vi "Read Search.vi"(11 "DiagramObject in":refnum<class "DiagramObject.lvclass">) -> (2 "Search":refnum<class "Search.lvclass">, 3 "DiagramObject out":refnum<class "DiagramObject.lvclass">)   [LabVIEW 2016, in "DiagramObject.lvclass"]
uses:
  DiagramObject.lvclass
  Search/Search.lvclass
  DiagramObject.lvclass/DiagramObject.ctl
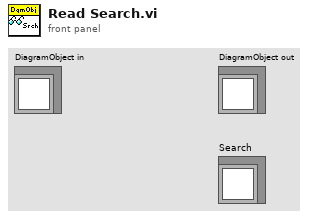
[diagram p1: front panel]
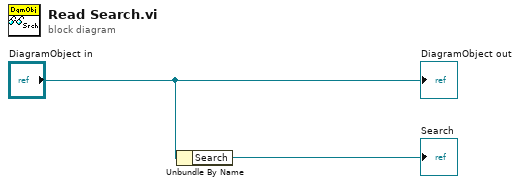
[diagram p0: block diagram]
diagram:
  n1 = Unbundle By Name("DiagramObject in") -> ("Search"=→"Search":refnum<class "Search.lvclass">)
  "DiagramObject out" <- "DiagramObject in"
